vi "STA - Wave V5 Host_Wait_V2.1.vi"() -> ()   [LabVIEW 2015]
doc: "The continuous acquisition mode tells the FPGA to acquire points indefinitely until a stop command is issued or until an error is encountered (FIFO overflow, module underflow, and so on). \n\nIn this acquisition mode, explicitly call the appropriate rwfm_ConfigTiming VI and set the host application's data buffer to be many times larger than the read size. The examples use a 10X size by default. If the host application's data buffer fills, then the FPGA experiences a FIFO overflow causing the acquisition to stop."
uses:
  <vilib>/LabVIEW Targets/FPGA/cRIO/shared/nicrio_ModuleControls/nicrio_cRIO-9234_ConfigModeRing.ctl
  <vilib>/Platform/TimedLoop/XDataNode/timing_clust.ctl
  <vilib>/Platform/TimedLoop/XDataNode/nitl_modes.ctl
  <vilib>/Platform/TimedLoop/XDataNode/wakeup.ctl
  <vilib>/FPGAPlugInAG/cRIO-9112/niLvFpga_Open_cRIO-9112.vi
  <vilib>/rvi/interface/common/dynamic/niFpgaDynamicAddResources.vi
  <vilib>/Utility/error.llb/Error Cluster From Error Code.vi
  <vilib>/RVI Host/nirviSupport.llb/nirviErrorClusterFromErrorCode.vi
  <vilib>/rvi/errors/niLvFpgaAdjustHostInterfaceError.vi
  <vilib>/FPGAPlugInAG/Dynamic/niLvFpga_Close_Dynamic.vi
  <vilib>/rvi/interface/nirviOpenFPGA/nirviOpenFPGA.xnode
  FPGA Bitfiles/STA-WaveformV5_FPGATarget2_[FPGA]DeltaSigMa_sLRIAVfzKK0.lvbitx
  FPGA/[FPGA] DeltaSig Main V5.vi
  <vilib>/rvi/interface/nirviMethod/nirviMethod.xnode
  <vilib>/rvi/interface/nirviCloseFPGA/nirviCloseFPGA.xnode
  <vilib>/Platform/TimedLoop/XDataNode/XDataNode.xnode
  <vilib>/NI/cRIO Wfm/cRIO Wfm.lvlib
  <vilib>/rvi/interface/nirviMethod/StockFPGA_InlinedMethodWaitForSingleIRQ.vi
  <vilib>/FPGAPlugInAG/Dynamic/niLvFpga_WaitOnIrq_Dynamic.vi
  C:/Program Files (x86)/National Instruments/LabVIEW 2015/ProjectTemplates/Source/cRIOWfm/FPGA/[FPGA] SAR Acq Main.vi
  D/Documents/LabVIEW Data/STA - Waveform V0/FPGA Bitfiles/SARAcqMain_9074.lvbitx
  <vilib>/Platform/TimedLoop/XDataNode/XDNodeRunTimeDep.lvlib
panel:
  out "Array 2":waveform(sgl)[](array[waveform])
  out "Size Waveform":i32
  out "size(s) 2":i32[](array[numeric])
  out "Y":sgl[][](array[numeric])
  in  "appended array 2":sgl[](array[numeric])
  out "appended array":sgl[](array[numeric])
  out "size(s)":i32[](array[numeric])
  out "i RT FIFO Read":i32
  out "Element 2":u32
  out "Element 1":u32
  out "transposed array":sgl[][](array[numeric])
  out "error out 2":errorcluster
  out "error out":errorcluster
  out "error fifo out":errorcluster
  out "Waveform Graph 2":sgl[][](graph)
  in  "Array":waveform(sgl)[](array[waveform])
  out "Waveform Graph":waveform(sgl)[](graph)
  out "Buffer Backlog":dbl caption="RT Buffer Backlog [%]" format="%#.2g"
  in  "Stop":bool
  in  "Amplitude":dbl(slide)=5.0 scale=0.0..10.0
  out "Time Measure":dbl
  out "data rate (S/s)":u32
  out "Channel Config":T2(array[cluster]) {"Input Configuration" items=["AC Coupled", "DC Coupled", "IEPE AC Coupled"]}
  in  "Samples per Read":i32=900
  # "Sampling Info"
  # "Channel Info"
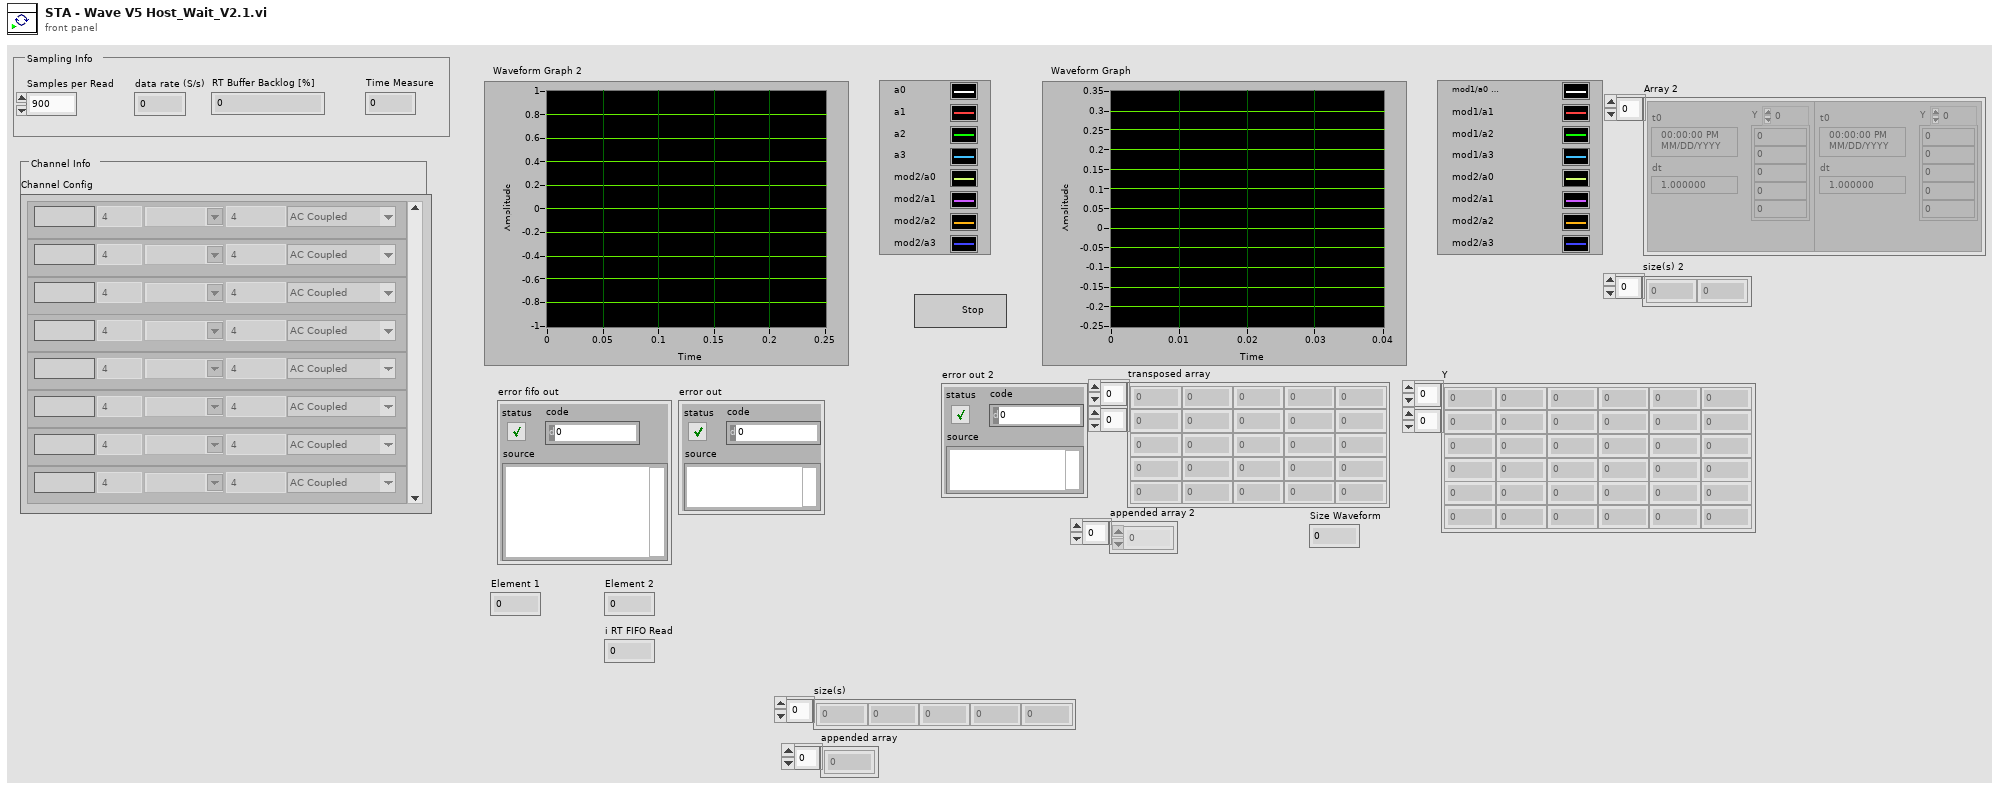
[diagram p1: front panel]
types:
  T1 = typedef "nicrio_cRIO-9234_ConfigModeRing.ctl" = u8
  T2 = cluster{"Channel Name":string, "Sensitivity mV_EU":dbl, "EU":string, "Input Configuration":T1, "dB Ref EU":dbl}[]
  T3 = typedef "XDNodeRunTimeDep.lvlib/timing_clust.ctl" = cluster{"Expected End [f-1]":u64, "Actual End [f-1]":u64, "Finished Late? [f-1]":bool, "Expected End [i-1]":u64, "Actual End [i-1]":u64, "Finished Late? [i-1]":bool, "Expected Start [i]":u64, "Actual Start [i]":u64, "Expected Start [f]":u64, "Actual Start [f]":u64, "Source Name":string, "Structure Name":string, "Period":i64, "Deadline":i64, "Offset":i64, "Start":i64, "Priority":i32, "Timeout":i32, "Mode":T4, "Wakeup Reason":T5, "Error":errorcluster, "Source Type":string, "Secondary Source Type":string, "Global End Time":u64, "Global Start Time":u64, "Frame Duration":u64, "Iteration Duration":u64, "Assigned CPU":i32, "I/O Scan Engine Mode":u32}
  T4 = typedef "XDNodeRunTimeDep.lvlib/nitl_modes.ctl" = enum32{"No Change", "Process missed periods, maintain original phase", "Discard missed periods, maintain original phase", "Process missed periods, ignore original phase", "Discard missed periods, ignore original phase"}
  T5 = typedef "XDNodeRunTimeDep.lvlib/wakeup.ctl" = enum32{"Normal", "Aborted", "Asynchronous wakeup", "Timing source error", "Timed loop error", "Timeout"}
  T6 = typedef "Acquisition and Logging Configuration_Waveform.ctl" = cluster{"Samples per Read":i32, "Number of Reads to Save":i32, "Data File Name":string, "TDMS Properties":T7[], "Number of Channels":i32, "Trigger - RMS Value":dbl, "Trigger - Channel":i32, "Trigger - Time (Minute)":i32, "Channel Config":cluster{"Channel Name":string, "Sensitivity mV_EU":dbl, "EU":string, "Input Configuration":T1, "dB Ref EU":dbl}[], "data rate (S/s)":u32, "Time Measure":dbl}
  T7 = typedef "TDMS Properties.ctl" = cluster{"Name":string, "Value":string}
  T8 = typedef "cRIO Wfm.lvlib/SamplingInfo.ctl" = cluster{"Number of Channels":i32, "Actual Samp Rate":dbl, "Chan Name Array":string[], "EU Chan Array":string[], "dB Ref Chan Array":dbl[]}
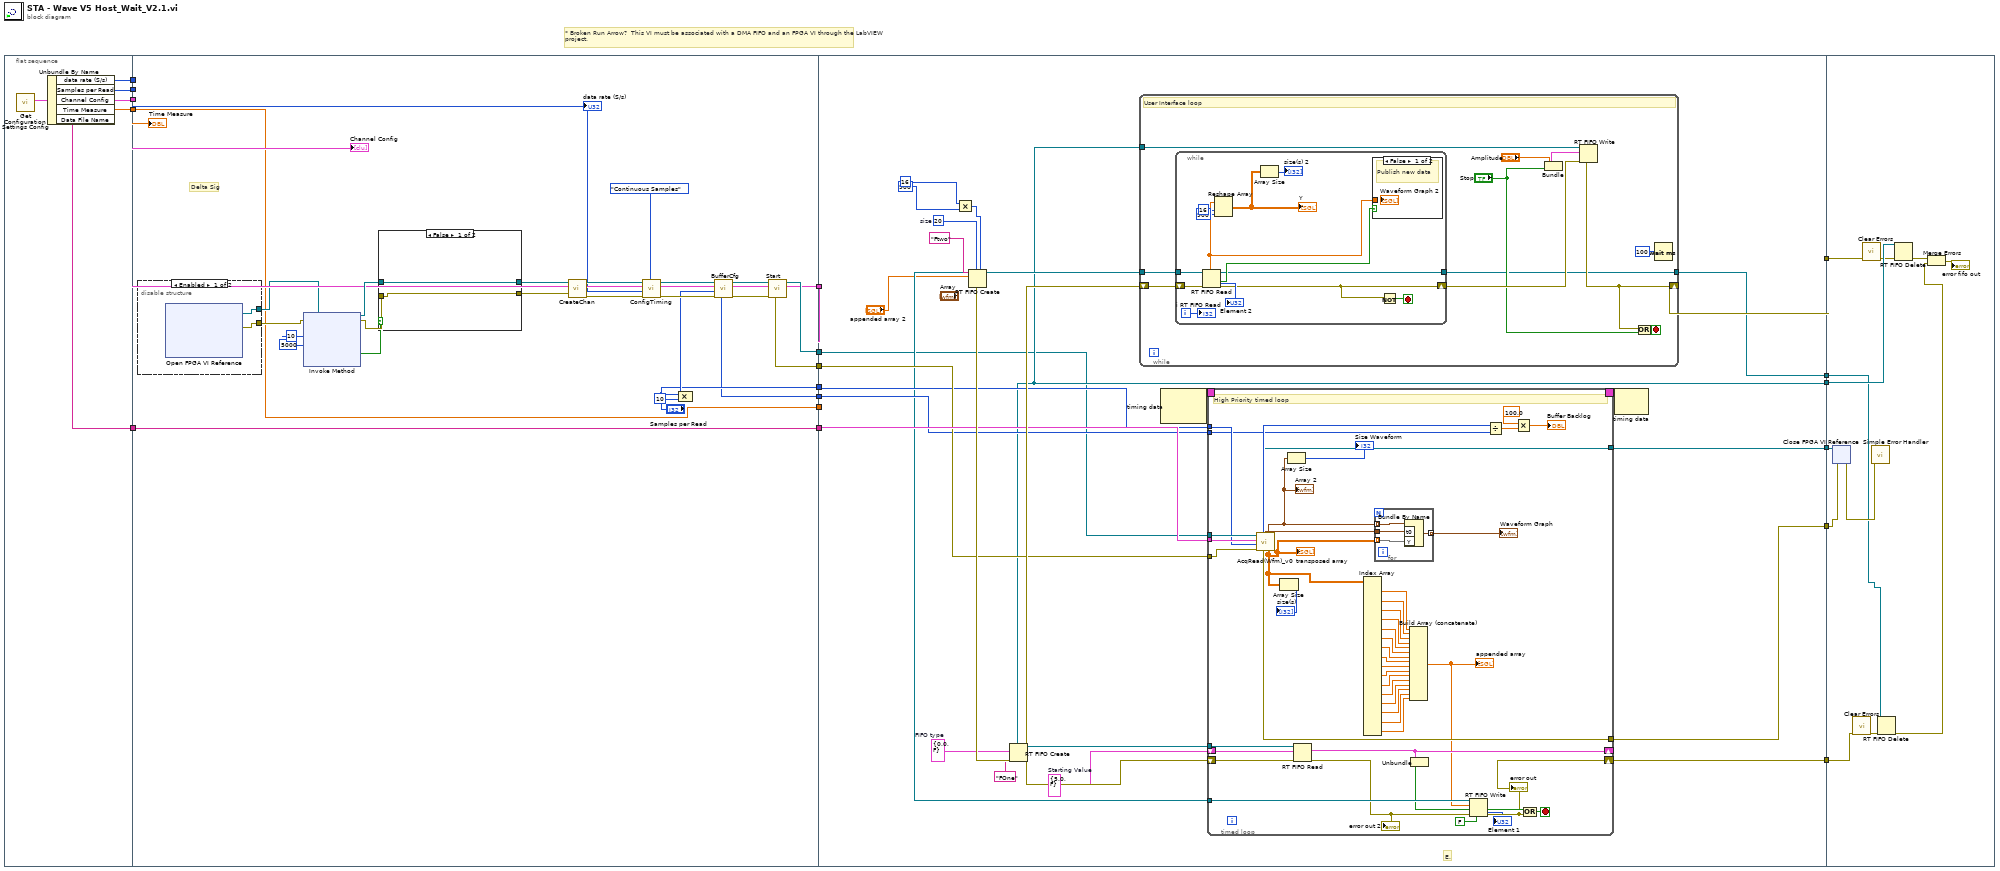
[diagram p0: block diagram]
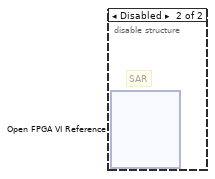
[diagram p2: hidden frame]
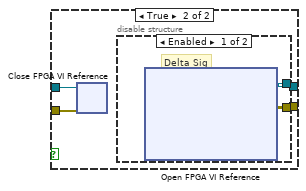
[diagram p3: hidden frame]
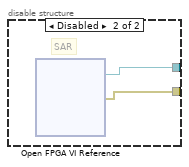
[diagram p4: hidden frame]
diagram:
  # "* Broken Run Arrow?  This VI must be associated with a DMA FIFO and an FPGA VI through the LabVIEW project."
  n1 = flat-sequence {
    tunnel: [w23] -> w18
    tunnel: [w22] -> w17
    tunnel: [w21] -> w16
    tunnel: [w20] -> w15
    tunnel: [w19] -> w8
    tunnel: w18 -> [w36]
    tunnel: w17 -> [_]
    tunnel: w16 -> [w35]
    tunnel: w15 -> [w28]
    tunnel: ["Samples per Read"] -> w14
    tunnel: [w28] -> w13
    tunnel: [w32] -> w12
    tunnel: [w31] -> w11
    tunnel: [w30] -> w10
    tunnel: [w27] -> w9
    tunnel: w8 -> [w26]
    tunnel: [w26] -> w7
    tunnel: w14 -> [w84]
    tunnel: w13 -> [_]
    tunnel: w12 -> [w74]
    tunnel: w11 -> [w86]
    tunnel: w10 -> [w85]
    tunnel: w9 -> [w83]
    tunnel: w7 -> [_]
    tunnel: [w81] -> w6
    tunnel: [w80] -> w5
    tunnel: [w79] -> w4
    tunnel: [w75] -> w3
    tunnel: [w77] -> w2
    tunnel: [w76] -> w1
    tunnel: w6 -> [w178]
    tunnel: w5 -> [w177]
    tunnel: w4 -> [w176]
    tunnel: w3 -> [w174]
    tunnel: w2 -> [w175]
    tunnel: w1 -> [w173]
    frame #0 {
      n2 = call "Get Configuration Settings Config.vi"() -> ("Configuration"=w24:T6)  [unwired: 10 in, 1 out]
      n3 = Unbundle By Name(w24) -> ("data rate (S/s)"=w23:u32, "Samples per Read"=w22:i32, "Channel Config"=w21:T2, "Time Measure"=w20:dbl, "Data File Name"=w19:string)
    }
    frame #1 {
      # "Delta Sig"
      n4 = disable-structure shown="Enabled" {
        disable-tunnel: [w56 _] -> w34
        disable-tunnel: [w55 _] -> w33
        frame Enabled {
          n5 = xnode "Open FPGA VI Reference"() -> ("FPGA VI Reference Out"=w56:refnum<k20>, "error out"=w55:errorcluster)  [unwired: 2 in]
        }
        frame Disabled {
          # "SAR"
          n6 = xnode "Open FPGA VI Reference"() -> ("FPGA VI Reference Out"=w58:refnum<k20>, "error out"=w57:errorcluster)  [unwired: 2 in]
        }
      }
      n7 = xnode "Invoke Method"("FPGA VI Reference In"=w34, "error in"=w33, "IRQ Number(s)"=10, "Timeout (ms)"=5000) -> ("FPGA VI Reference Out"=w52:refnum<k20>, "error out"=w53:errorcluster, "Timed Out"=w51:bool)  [unwired: 1 out]
      n8 = case shown="False" w51 {
        tunnel: w52 -> [w60 w64]
        tunnel: w53 -> [w59 w63]
        tunnel: [w60 w62] -> w25
        tunnel: [w59 w61] -> w54
        frame False {
        }
        frame True {
          n9 = xnode "Close FPGA VI Reference"("FPGA VI Reference In"=w64, "error in"=w63) -> ()  [unwired: 1 out]
          n10 = disable-structure shown="Enabled" {
            disable-tunnel: [w66 w68] -> w62
            disable-tunnel: [w65 w67] -> w61
            frame Enabled {
              # "Delta Sig"
              n11 = xnode "Open FPGA VI Reference"() -> ("FPGA VI Reference Out"=w66:refnum<k20>, "error out"=w65:errorcluster)  [unwired: 2 in]
            }
            frame Disabled {
              # "SAR"
              n12 = xnode "Open FPGA VI Reference"() -> ("FPGA VI Reference Out"=w68:refnum<k20>, "error out"=w67:errorcluster)  [unwired: 2 in]
            }
          }
        }
      }
      n13 = call <vilib>:"CreateChan.vi"("Dynamic FPGA Ref"=w25, "Channel Config"=w35, "error in"=w54) -> ("Dynamic FPGA Ref Out"=w42:refnum<k20>, "Sampling Info"=w43:T8, "error out"=w47:errorcluster)  [unwired: 5 in]
      n14 = call <vilib>:"ConfigTiming.vi"("Sample Mode"=enum16{"Finite Samples", "Continuous Samples"}."Continuous Samples", "error in"=w47, "Sample Rate"=w36, "Sampling Info In"=w43, "Dynamic FPGA Ref"=w42) -> ("error out"=w46:errorcluster, "Sampling Info Out"=w45:T8, "Dynamic FPGA Ref Out"=w44:refnum<k20>)  [unwired: 3 in, 1 out]
      n15 = Compound Arithmetic op=MULTIPLY("Samples per Read", 10 ("value")) -> (w40:i32)
      n16 = call <vilib>:"BufferCfg.vi"("error in"=w46, "Buffer Size [Samps per Chan]"=w40, "Sampling Info In"=w45, "Dynamic FPGA Ref"=w44) -> ("error out"=w39:errorcluster, "Buffer Size [Total Samples]"=w27:u32, "Sampling Info Out"=w41:T8, "Dynamic FPGA Ref Out"=w38:refnum<k20>)  [unwired: 4 out]
      n17 = call <vilib>:"Start.vi"("error in"=w39, "Sampling Info In"=w41, "Dynamic FPGA Ref"=w38) -> ("error out"=w30:errorcluster, "Sampling Info Out"=w31:T8, "Dynamic FPGA Ref Out"=w32:refnum<k20>)  [unwired: 6 out]
      "Channel Config" <- w35
      "data rate (S/s)" <- w36
      "Time Measure" <- w28
    }
    frame #2 {
      w87 = cluster{dbl, bool} {5.0, FALSE}  # Starting Value
      w88 = cluster{dbl, bool} {0.0, FALSE}  # FIFO type
      w89 = u32 20  # size
      # "E."
      n18 = Multiply(x=16 ("dimension size"), y=900 ("dimension size")) -> (x*y=w71:i32)
      n19 = RT FIFO Create(0:"Ftwo" ("name (unnamed)"), 1:"appended array 2", 4:w89, 6:w71) -> (8:w78:refnum<k33>, 11:w91:errorcluster)  [unwired: 2 in, 3 out]
      n20 = RT FIFO Create(0:"FOne" ("name (unnamed)"), 1:w88, 3:w91) -> (8:w77:refnum<k33>, 11:w90:errorcluster)  [unwired: 2 in, 4 out]
      n21 = while "User Interface loop" {
        shift-right: [w147] -> w76
        shift-left: w90 -> [w155]
        tunnel: w77 -> [w154]
        tunnel: w78 -> [w156]
        tunnel: [w146] -> w75
        stop <- w152 stop-if-true
        # "User Interface loop"
        n22 = while {
          tunnel: w156 -> [w169]
          shift-right: [w162] -> w153
          shift-left: w155 -> [w168]
          tunnel: [w165] -> w146
          i -> [w164]
          stop <- w163 stop-if-true
          n23 = RT FIFO Read(0:w169, 3:w168) -> (7:→"Element 2":u32, 8:w165:refnum<k33>, 9:w161:sgl[], 10:w167:bool, 11:w162:errorcluster)  [unwired: 1 in, 1 out]
          n24 = Reshape Array(w161, 16 ("dimension size"), 900 ("dimension size")) -> (w158:sgl[][])
          "Y" <- w158
          n25 = Array Size(array=w158) -> (size(s)=→"size(s) 2":i32[])
          n26 = case shown="False" w167 {
            tunnel: w161 -> [_ _]
            frame False {
              # "Publish new data"
            }
            frame True {
              # "No new data"
            }
          }
          n27 = Not(x=w162) -> (.not. x?=w163:bool)
          "i RT FIFO Read" <- w164
        }
        n28 = Bundle("Amplitude"="Amplitude", "Stop"="Stop") -> (w149:cluster{"Amplitude":dbl, "Stop":bool})  [unwired: 1 in]
        n29 = RT FIFO Write(0:w154, 1:w149, 3:w153) -> (11:w147:errorcluster)  [unwired: 2 in, 3 out]
        n30 = Or(x=w147, y="Stop") -> (x .or. y?=w152:bool)
        n31 = Wait (ms)(milliseconds to wait=u32 100 ("millisecond multiple")) -> ()  [unwired: 1 out]
      }
      n32 = node-c288() -> (w93:T3)  [unwired: 1 in, 1 out]
      n33 = timed-loop "High Priority timed loop" {
        shift-left: w87 -> [w137]
        shift-right: [w133] -> _
        shift-right: [w117] -> w79
        shift-left: w90 -> [w134]
        timing: w93 -> [_]
        timing-out: [_] -> w92
        tunnel: w77 -> [w138]
        tunnel: w78 -> [w136]
        tunnel: w86 -> [w125]
        tunnel: w74 -> [w124]
        tunnel: w85 -> [w123]
        tunnel: w84 -> [w122]
        tunnel: w83 -> [w121]
        tunnel: [w119] -> w81
        tunnel: [w118] -> w80
        stop <- w131 stop-if-true
        # "High Priority timed loop"
        n34 = call <vilib>:"AcqRead(Wfm)_v0.vi"("error in"=w123, "Samps Read per Chan"=w122, "Sampling Info"=w125, "Dynamic FPGA Ref"=w124) -> ("error out"=w118:errorcluster, "Samples Remaining"=w130:u32, "time stamp"=w126:timestamp, "Dynamic FPGA Ref Out"=w119:refnum<k20>, "transposed array"=w113:sgl[][], "Array"=w95:waveform(sgl)[])  [unwired: 2 in]
        "transposed array" <- w113
        "Array 2" <- w95
        n35 = Array Size(array=w113) -> (size(s)=→"size(s)":i32[])
        n36 = Array Size(array=w95) -> (size(s)=→"Size Waveform":i32)
        n37 = RT FIFO Read(0:w138, 1:w137, 3:w134) -> (9:w133:cluster{dbl, bool}, 11:w135:errorcluster)  [unwired: 4 out]
        "error out 2" <- w135
        n38 = Index Array(array=w113) -> (element #1=w112:sgl[], element #2=w111:sgl[], element #3=w110:sgl[], element #4=w109:sgl[], element #5=w108:sgl[], element #6=w107:sgl[], element #7=w106:sgl[], element #8=w105:sgl[], element #9=w104:sgl[], element #10=w103:sgl[], element #11=w102:sgl[], element #12=w101:sgl[], element #13=w100:sgl[], element #14=w99:sgl[], element #15=w98:sgl[], element #16=w97:sgl[])  [unwired: 32 in]
        n39 = for {
          tunnel: w95 -> [w142] mode=indexing
          tunnel: w126 -> [w141]
          tunnel: [w140] -> w120 mode=indexing
          tunnel: w113 -> [w139] mode=indexing
          n40 = Bundle By Name(cluster=w142, "t0"=w141, "Y"=w139) -> (w140:waveform(sgl))
        }
        "Waveform Graph" <- w120
        n41 = Build Array (concatenate)(w112, w111, w110, w109, w108, w107, w106, w105, w104, w103, w102, w101, w100, w99, w98, w97) -> (w96:sgl[])
        "appended array" <- w96
        n42 = Unbundle(w133) -> (w132:bool)  [unwired: 1 out]
        n43 = RT FIFO Write(0:w136, 1:w96, 3:w135, 5:FALSE ("overwrite on timeout (T)")) -> (7:→"Element 1":u32, 11:w117:errorcluster)  [unwired: 3 out]
        "error out" <- w117
        n44 = Divide(x=w130, y=w121) -> (x/y=w129:dbl)
        n45 = Multiply(x=100.0, y=w129) -> (x*y=→"Buffer Backlog":dbl)
        n46 = Or(x=w132, y=w117) -> (x .or. y?=w131:bool)
      }
      n47 = node-c288(w92) -> ()  [unwired: 1 out]
    }
    frame #3 {
      n48 = xnode "Close FPGA VI Reference"("FPGA VI Reference In"=w178, "error in"=w177) -> ("error out"=w182:errorcluster)
      n49 = call <vilib>:"Clear Errors.vi"("error in (no error)"=w176) -> ("error out"=w179:errorcluster)  [unwired: 5 in, 1 out]
      n50 = call <vilib>:"Clear Errors.vi"("error in (no error)"=w173) -> ("error out"=w172:errorcluster)  [unwired: 5 in, 1 out]
      n51 = call <vilib>:"Simple Error Handler.vi"("error in (no error)"=w182) -> ()  [unwired: 1 in, 8 out]
      n52 = RT FIFO Delete(0:w174, 3:w179) -> (11:w171:errorcluster)  [unwired: 1 in]
      n53 = RT FIFO Delete(0:w175, 3:w172) -> (11:w180:errorcluster)  [unwired: 1 in]
      n54 = Merge Errors(w180, w171) -> (→"error fifo out":errorcluster)
    }
  }
